vi "New Mixer Trace.vi"(0 "VISA IN":refnum<visa-resource-name>, 1 "Meas Param":string(combo)="S21", 2 "FileName":string="Test", 3 "Window":i32=1, 4 "Trace":i32=2, 5 "error in (no error)":errorcluster, 6 "Meas Type":string="Test", 7 "Channel":i32=1) -> (14 "VISA Out":refnum<visa-resource-name>, 19 "error out":errorcluster)   [LabVIEW 2018, in "PNA-X.lvlib"]
uses:
  PNA-X.lvlib
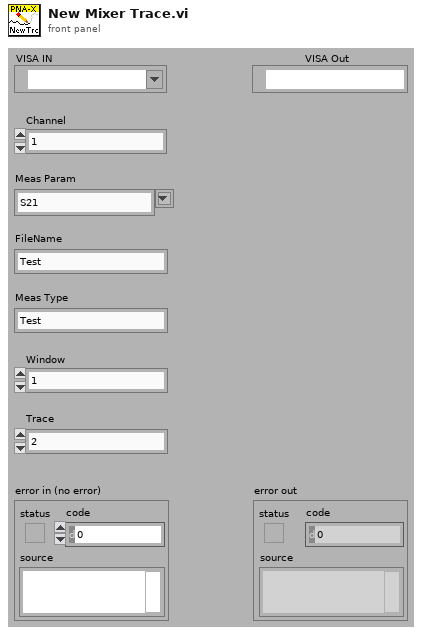
[diagram p1: front panel]
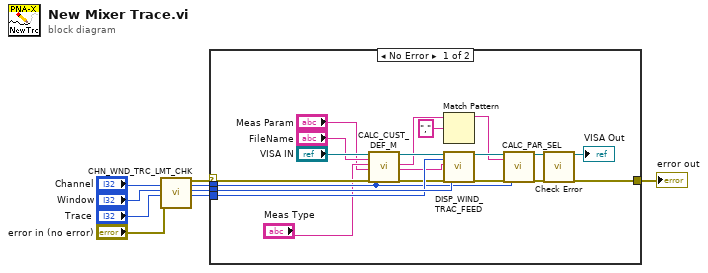
[diagram p0: block diagram]
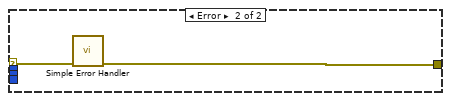
[diagram p2: hidden frame]
diagram:
  n1 = call "CHN_WND_TRC_LMT_CHK.vi"("Channel"="Channel", "Window"="Window", "Trace"="Trace", "error in"="error in (no error)") -> ("error out"=w8:errorcluster, "Channel"=w3:i32, "Window"=w2:i32, "Trace"=w1:i32)  [unwired: 11 in, 1 out]
  n2 = case shown="No Error" w8 {
    selector: w8 -> [w20 w31]
    tunnel: [w29 w30] -> w9
    tunnel: w3 -> [w16 _]
    tunnel: w2 -> [w22 _]
    tunnel: w1 -> [w21 _]
    frame No Error {
      n3 = call "CALC_CUST_DEF_M.vi"("VISA IN"="VISA IN", "Measurement Name"="FileName", "Measurement Type"="Meas Type", "Measurement Parameter"="Meas Param", "error in"=w20, "Channel"=w16) -> ("VISA Out"=w17:refnum<visa-resource-name>, "Meas"=w15:string, "Filename"=w11:string, "error out"=w19:errorcluster)  [unwired: 10 in]
      n4 = Match Pattern(string=w15, regular expression=",") -> (before substring=w10:string)  [unwired: 1 in, 3 out]
      n5 = call "DISP_WIND_TRAC_FEED.vi"("VISA IN"=w17, "Trace"=w21, "Name"=w11, "error in"=w19, "Window"=w22) -> ("VISA Out"=w24:refnum<visa-resource-name>, "error out"=w23:errorcluster)  [unwired: 13 in]
      n6 = call "CALC_PAR_SEL.vi"("VISA IN"=w24, "Measurement"=w10, "error in"=w23, "Channel"=w16) -> ("VISA Out"=w25:refnum<visa-resource-name>, "error out"=w27:errorcluster)  [unwired: 14 in]
      n7 = call "Check Error.vi"("VISA Resource Name"=w25, "error in (no error)"=w27) -> ("dup VISA session"=→"VISA Out":refnum<visa-resource-name>, "error out"=w29:errorcluster)  [unwired: 16 in]
    }
    frame Error {
      n8 = call <vilib>:"Simple Error Handler.vi"("error in (no error)"=w31) -> ("error out"=w30:errorcluster)  [unwired: 4 in, 4 out]
    }
  }
  "error out" <- w9
